vi "ParseSlaveRY.vi"(0 "RY":bool[][](array[boolean])) -> (1 "PLC状态":T2, 2 "检测步骤":T3)   [LabVIEW 2018]
panel:
  out "PLC结果":T1
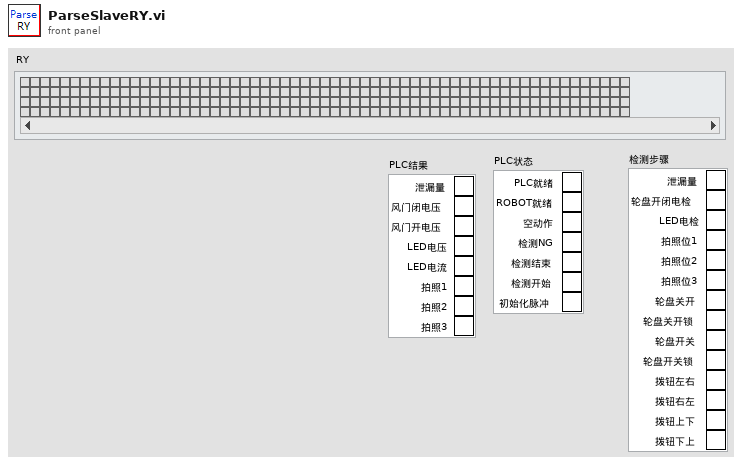
[diagram p1: front panel]
types:
  T1 = cluster{"泄漏量":bool, "风门闭电压":bool, "风门开电压":bool, "LED电压":bool, "LED电流":bool, "拍照1":bool, "拍照2":bool, "拍照3":bool}
  T2 = cluster{"PLC就绪":bool, "ROBOT就绪":bool, "空动作":bool, "检测NG":bool, "检测结束":bool, "检测开始":bool, "初始化脉冲":bool}
  T3 = cluster{"泄漏量":bool, "轮盘开闭电检":bool, "LED电检":bool, "拍照位1":bool, "拍照位2":bool, "拍照位3":bool, "轮盘关开":bool, "轮盘关开锁":bool, "轮盘开关":bool, "轮盘开关锁":bool, "拨钮左右":bool, "拨钮右左":bool, "拨钮上下":bool, "拨钮下上":bool}
  T4 = cluster{"泄漏量":bool, "风门开闭电检":bool, "LED电检":bool, "拍照位1":bool, "拍照位2":bool, "拍照位3":bool, "轮盘关开":bool, "轮盘关开锁":bool, "轮盘开关":bool, "轮盘开关锁":bool, "拨钮左右":bool, "拨钮右左":bool, "拨钮上下":bool, "拨钮下上":bool}
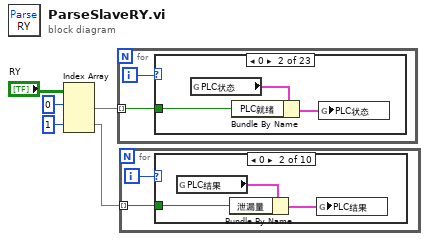
[diagram p0: block diagram]
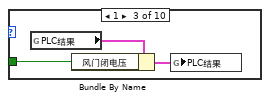
[diagram p3: hidden frame]
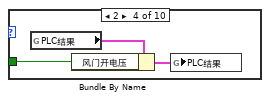
[diagram p4: hidden frame]
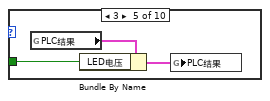
[diagram p5: hidden frame]
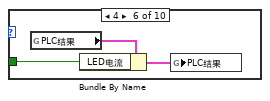
[diagram p6: hidden frame]
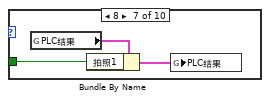
[diagram p7: hidden frame]
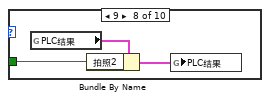
[diagram p8: hidden frame]
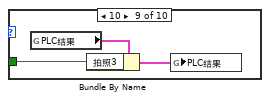
[diagram p9: hidden frame]
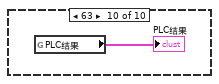
[diagram p10: hidden frame]
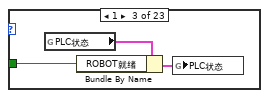
[diagram p12: hidden frame]
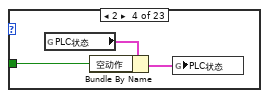
[diagram p13: hidden frame]
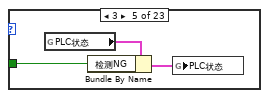
[diagram p14: hidden frame]
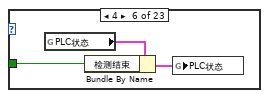
[diagram p15: hidden frame]
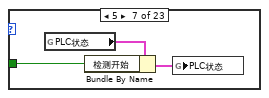
[diagram p16: hidden frame]
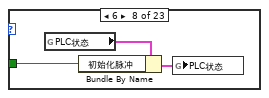
[diagram p17: hidden frame]
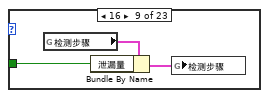
[diagram p18: hidden frame]
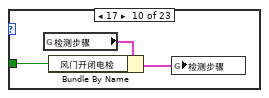
[diagram p19: hidden frame]
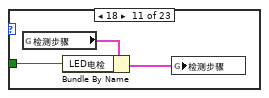
[diagram p20: hidden frame]
diagram:
  n1 = Index Array(array="RY", index (row) #1=0 ("索引 (行)"), index (row) #2=1 ("索引 (行)")) -> (element #1=w3:bool[], element #2=w1:bool[])  [unwired: 2 in]
  n2 = for {
    tunnel: w3 -> [w6] mode=indexing
    i -> [w7]
    n3 = case shown="0" w7 {
      tunnel: w6 -> [_ w9 w12 w15 w18 w21 w24 w27 w30 w33 w36 w39 w42 w45 w48 w51 w54 w57 w60 w63 w66 w69 _]
      frame -1, Default {
      }
      frame 0 {
        n4 = global read "全局 1.vi" "PLC状态"() -> (w10:T2)
        n5 = Bundle By Name(cluster=w10, "PLC就绪"=w9) -> (w8:T2)
        n6 = global write "全局 1.vi" "PLC状态"(w8) -> ()
      }
      frame 1 {
        n7 = global read "全局 1.vi" "PLC状态"() -> (w13:T2)
        n8 = Bundle By Name(cluster=w13, "ROBOT就绪"=w12) -> (w11:T2)
        n9 = global write "全局 1.vi" "PLC状态"(w11) -> ()
      }
      frame 2 {
        n10 = global read "全局 1.vi" "PLC状态"() -> (w16:T2)
        n11 = Bundle By Name(cluster=w16, "空动作"=w15) -> (w14:T2)
        n12 = global write "全局 1.vi" "PLC状态"(w14) -> ()
      }
      frame 3 {
        n13 = global read "全局 1.vi" "PLC状态"() -> (w19:T2)
        n14 = Bundle By Name(cluster=w19, "检测NG"=w18) -> (w17:T2)
        n15 = global write "全局 1.vi" "PLC状态"(w17) -> ()
      }
      frame 4 {
        n16 = global read "全局 1.vi" "PLC状态"() -> (w22:T2)
        n17 = Bundle By Name(cluster=w22, "检测结束"=w21) -> (w20:T2)
        n18 = global write "全局 1.vi" "PLC状态"(w20) -> ()
      }
      frame 5 {
        n19 = global read "全局 1.vi" "PLC状态"() -> (w25:T2)
        n20 = Bundle By Name(cluster=w25, "检测开始"=w24) -> (w23:T2)
        n21 = global write "全局 1.vi" "PLC状态"(w23) -> ()
      }
      frame 6 {
        n22 = global read "全局 1.vi" "PLC状态"() -> (w28:T2)
        n23 = Bundle By Name(cluster=w28, "初始化脉冲"=w27) -> (w26:T2)
        n24 = global write "全局 1.vi" "PLC状态"(w26) -> ()
      }
      frame 16 {
        n25 = global read "全局 1.vi" "检测步骤"() -> (w31:T4)
        n26 = Bundle By Name(cluster=w31, "泄漏量"=w30) -> (w29:T4)
        n27 = global write "全局 1.vi" "检测步骤"(w29) -> ()
      }
      frame 17 {
        n28 = global read "全局 1.vi" "检测步骤"() -> (w34:T4)
        n29 = Bundle By Name(cluster=w34, "风门开闭电检"=w33) -> (w32:T4)
        n30 = global write "全局 1.vi" "检测步骤"(w32) -> ()
      }
      frame 18 {
        n31 = global read "全局 1.vi" "检测步骤"() -> (w37:T4)
        n32 = Bundle By Name(cluster=w37, "LED电检"=w36) -> (w35:T4)
        n33 = global write "全局 1.vi" "检测步骤"(w35) -> ()
      }
      frame 25 {
        n34 = global read "全局 1.vi" "检测步骤"() -> (w40:T4)
        n35 = Bundle By Name(cluster=w40, "拍照位1"=w39) -> (w38:T4)
        n36 = global write "全局 1.vi" "检测步骤"(w38) -> ()
      }
      frame 26 {
        n37 = global read "全局 1.vi" "检测步骤"() -> (w43:T4)
        n38 = Bundle By Name(cluster=w43, "拍照位2"=w42) -> (w41:T4)
        n39 = global write "全局 1.vi" "检测步骤"(w41) -> ()
      }
      frame 27 {
        n40 = global read "全局 1.vi" "检测步骤"() -> (w46:T4)
        n41 = Bundle By Name(cluster=w46, "拍照位3"=w45) -> (w44:T4)
        n42 = global write "全局 1.vi" "检测步骤"(w44) -> ()
      }
      frame 32 {
        n43 = global read "全局 1.vi" "检测步骤"() -> (w49:T4)
        n44 = Bundle By Name(cluster=w49, "轮盘关开"=w48) -> (w47:T4)
        n45 = global write "全局 1.vi" "检测步骤"(w47) -> ()
      }
      frame 33 {
        n46 = global read "全局 1.vi" "检测步骤"() -> (w52:T4)
        n47 = Bundle By Name(cluster=w52, "轮盘关开锁"=w51) -> (w50:T4)
        n48 = global write "全局 1.vi" "检测步骤"(w50) -> ()
      }
      frame 34 {
        n49 = global read "全局 1.vi" "检测步骤"() -> (w55:T4)
        n50 = Bundle By Name(cluster=w55, "轮盘开关"=w54) -> (w53:T4)
        n51 = global write "全局 1.vi" "检测步骤"(w53) -> ()
      }
      frame 35 {
        n52 = global read "全局 1.vi" "检测步骤"() -> (w58:T4)
        n53 = Bundle By Name(cluster=w58, "轮盘开关锁"=w57) -> (w56:T4)
        n54 = global write "全局 1.vi" "检测步骤"(w56) -> ()
      }
      frame 36 {
        n55 = global read "全局 1.vi" "检测步骤"() -> (w61:T4)
        n56 = Bundle By Name(cluster=w61, "拨钮左右"=w60) -> (w59:T4)
        n57 = global write "全局 1.vi" "检测步骤"(w59) -> ()
      }
      frame 37 {
        n58 = global read "全局 1.vi" "检测步骤"() -> (w64:T4)
        n59 = Bundle By Name(cluster=w64, "拨钮右左"=w63) -> (w62:T4)
        n60 = global write "全局 1.vi" "检测步骤"(w62) -> ()
      }
      frame 38 {
        n61 = global read "全局 1.vi" "检测步骤"() -> (w67:T4)
        n62 = Bundle By Name(cluster=w67, "拨钮上下"=w66) -> (w65:T4)
        n63 = global write "全局 1.vi" "检测步骤"(w65) -> ()
      }
      frame 39 {
        n64 = global read "全局 1.vi" "检测步骤"() -> (w70:T4)
        n65 = Bundle By Name(cluster=w70, "拨钮下上"=w69) -> (w68:T4)
        n66 = global write "全局 1.vi" "检测步骤"(w68) -> ()
      }
      frame 63 {
        n67 = global read "全局 1.vi" "检测步骤"() -> (→"检测步骤":T4)
        n68 = global read "全局 1.vi" "PLC状态"() -> (→"PLC状态":T2)
      }
    }
  }
  n69 = for {
    tunnel: w1 -> [w73] mode=indexing
    i -> [w74]
    n70 = case shown="0" w74 {
      tunnel: w73 -> [_ w75 w78 w81 w84 w87 w90 w93 w96 _]
      frame -1, Default {
      }
      frame 0 {
        n71 = global read "全局 1.vi" "PLC结果"() -> (w77:T1)
        n72 = Bundle By Name(cluster=w77, "泄漏量"=w75) -> (w76:T1)
        n73 = global write "全局 1.vi" "PLC结果"(w76) -> ()
      }
      frame 1 {
        n74 = global read "全局 1.vi" "PLC结果"() -> (w80:T1)
        n75 = Bundle By Name(cluster=w80, "风门闭电压"=w78) -> (w79:T1)
        n76 = global write "全局 1.vi" "PLC结果"(w79) -> ()
      }
      frame 2 {
        n77 = global read "全局 1.vi" "PLC结果"() -> (w83:T1)
        n78 = Bundle By Name(cluster=w83, "风门开电压"=w81) -> (w82:T1)
        n79 = global write "全局 1.vi" "PLC结果"(w82) -> ()
      }
      frame 3 {
        n80 = global read "全局 1.vi" "PLC结果"() -> (w86:T1)
        n81 = Bundle By Name(cluster=w86, "LED电压"=w84) -> (w85:T1)
        n82 = global write "全局 1.vi" "PLC结果"(w85) -> ()
      }
      frame 4 {
        n83 = global read "全局 1.vi" "PLC结果"() -> (w89:T1)
        n84 = Bundle By Name(cluster=w89, "LED电流"=w87) -> (w88:T1)
        n85 = global write "全局 1.vi" "PLC结果"(w88) -> ()
      }
      frame 8 {
        n86 = global read "全局 1.vi" "PLC结果"() -> (w92:T1)
        n87 = Bundle By Name(cluster=w92, "拍照1"=w90) -> (w91:T1)
        n88 = global write "全局 1.vi" "PLC结果"(w91) -> ()
      }
      frame 9 {
        n89 = global read "全局 1.vi" "PLC结果"() -> (w95:T1)
        n90 = Bundle By Name(cluster=w95, "拍照2"=w93) -> (w94:T1)
        n91 = global write "全局 1.vi" "PLC结果"(w94) -> ()
      }
      frame 10 {
        n92 = global read "全局 1.vi" "PLC结果"() -> (w98:T1)
        n93 = Bundle By Name(cluster=w98, "拍照3"=w96) -> (w97:T1)
        n94 = global write "全局 1.vi" "PLC结果"(w97) -> ()
      }
      frame 63 {
        n95 = global read "全局 1.vi" "PLC结果"() -> (→"PLC结果":T1)
      }
    }
  }
